vi "Task Init.vi"(8 "error in (no error)":errorcluster, 11 "DaqControl in":refnum<class "DaqControl.lvclass">) -> (0 "error out":errorcluster, 3 "DaqControl out":refnum<class "DaqControl.lvclass">)   [LabVIEW 2020, in "VolatusDaq.lvlib" / "DaqControl.lvclass"]
uses:
  DaqControl.lvclass
  DaqControl.lvclass/DaqControl.ctl
  Value Update.ctl
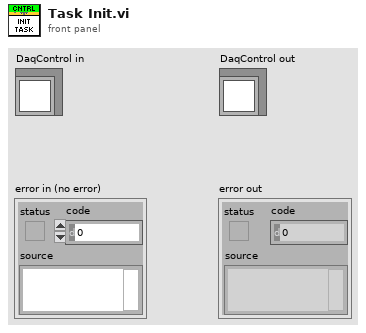
[diagram p1: front panel]
types:
  T1 = typedef "VolatusDaq.lvlib/DaqControl.lvclass/Value Update.ctl" = cluster{"Index":i32, "Value":dbl}
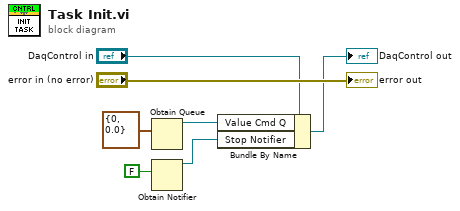
[diagram p0: block diagram]
diagram:
  n1 = Obtain Queue(element data type=T1 {"Index"=0, "Value"=0.0} ("Value Update")) -> (queue out=w3:refnum<queue>)  [unwired: 4 in, 2 out]
  n2 = Obtain Notifier(notification data type=FALSE) -> (notifier out=w1:refnum<notifier>)  [unwired: 3 in, 2 out]
  n3 = Bundle By Name(cluster="DaqControl in", "Value Cmd Q"=w3, "Stop Notifier"=w1) -> (→"DaqControl out":refnum<class "DaqControl.lvclass">)
  "error out" <- "error in (no error)"
